vi "getTagfromId.vi"(10 "ID":dbl, 11 "PipelineResult":T7={"TargetCount"=0, "Latency_MilliSec"=0.0, "Targets"=[], "TimeStampSec"=0.0, "PhotonMultiTargetPNPResult"={"PhotonPNPResult"={"IsPresent"=FALSE, "bestReprojErr"=0.0, "altReprojErr"=0.0, "ambiguity"=0.0, "Best"={"TRANSLATION3D"={"X"=0.0, "Y"=0.0, "Z"=0.0}, "ROTATION3D"={"Q_quaternion"={"R"=1.0, "V"=[0.0, 0.0, 0.0]}}, "XF"=FALSE}, "Alt"={"TRANSLATION3D"={"X"=0.0, "Y"=0.0, "Z"=0.0}, "ROTATION3D"={"Q_quaternion"={"R"=1.0, "V"=[0.0, 0.0, 0.0]}}, "XF"=FALSE}}, "FiducialIDsUsed"=[]}} {"PhotonMultiTargetPNPResult"."PhotonPNPResult"."Alt"."TRANSLATION3D"."Z" format="%14.3f"; "PhotonMultiTargetPNPResult"."PhotonPNPResult"."Alt"."TRANSLATION3D"."Y" format="%14.3f"; "PhotonMultiTargetPNPResult"."PhotonPNPResult"."Alt"."TRANSLATION3D"."X" format="%14.3f"; "PhotonMultiTargetPNPResult"."PhotonPNPResult"."Best"."TRANSLATION3D"."Z" format="%14.3f"; "PhotonMultiTargetPNPResult"."PhotonPNPResult"."Best"."TRANSLATION3D"."Y" format="%14.3f"; "PhotonMultiTargetPNPResult"."PhotonPNPResult"."Best"."TRANSLATION3D"."X" format="%14.3f"; "Targets"."AltCameraToTarget"."TRANSLATION3D"."Z" format="%14.3f"; "Targets"."AltCameraToTarget"."TRANSLATION3D"."Y" format="%14.3f"; "Targets"."AltCameraToTarget"."TRANSLATION3D"."X" format="%14.3f"; "Targets"."BestCameraToTarget"."TRANSLATION3D"."Z" format="%14.3f"; "Targets"."BestCameraToTarget"."TRANSLATION3D"."Y" format="%14.3f"; "Targets"."BestCameraToTarget"."TRANSLATION3D"."X" format="%14.3f"}) -> (3 "PhotonTrackedTarget":T1={"Yaw"=0.0, "Pitch"=0.0, "Area"=0.0, "Skew"=0.0, "MinAreaRectCorners"=[], "BestCameraToTarget"={"TRANSLATION3D"={"X"=0.0, "Y"=0.0, "Z"=0.0}, "ROTATION3D"={"Q_quaternion"={"R"=1.0, "V"=[0.0, 0.0, 0.0]}}, "XF"=FALSE}, "FiiducialId"=0, "AltCameraToTarget"={"TRANSLATION3D"={"X"=0.0, "Y"=0.0, "Z"=0.0}, "ROTATION3D"={"Q_quaternion"={"R"=1.0, "V"=[0.0, 0.0, 0.0]}}, "XF"=FALSE}, "PoseAmbiguity"=0.0, "DetectedCorners"=[]} {"AltCameraToTarget"."TRANSLATION3D"."Z" format="%14.3f"; "AltCameraToTarget"."TRANSLATION3D"."Y" format="%14.3f"; "AltCameraToTarget"."TRANSLATION3D"."X" format="%14.3f"; "BestCameraToTarget"."TRANSLATION3D"."Z" format="%14.3f"; "BestCameraToTarget"."TRANSLATION3D"."Y" format="%14.3f"; "BestCameraToTarget"."TRANSLATION3D"."X" format="%14.3f"})   [LabVIEW 2023]
uses:
  <vilib>/Rock Robotics/WPI/ThirdParty/PhotonVisionLib/TypeDef/PhotonPipelineResultType.ctl
  <vilib>/Rock Robotics/WPI/ThirdParty/PhotonVisionLib/TypeDef/PhotonTrackedTargetType.ctl
  <vilib>/Rock Robotics/WPI/ThirdParty/PhotonVisionLib/TypeDef/TargetCornerType.ctl
  <vilib>/Rock Robotics/WPI/ThirdParty/JAS_Junk/TrajLib/TypeDef/TRANSFORM3D.ctl
  <vilib>/Rock Robotics/WPI/ThirdParty/JAS_Junk/TrajLib/TypeDef/TRANSLATION3D.ctl
  <vilib>/Rock Robotics/WPI/ThirdParty/JAS_Junk/TrajLib/TypeDef/ROTATION3D.ctl
  <vilib>/Rock Robotics/WPI/ThirdParty/JAS_Junk/TrajLib/TypeDef/QUATERNION.ctl
  <vilib>/Rock Robotics/WPI/ThirdParty/PhotonVisionLib/TypeDef/PhotonMultiTargetPNPResultType.ctl
  <vilib>/Rock Robotics/WPI/ThirdParty/PhotonVisionLib/TypeDef/PhotonPNPResultType.ctl
  <vilib>/Rock Robotics/WPI/ThirdParty/PhotonVisionLib/PhotonVisionLib.lvlib
  <vilib>/Rock Robotics/WPI/ThirdParty/JAS_Junk/TrajLib/Trajectory_Library.lvlib
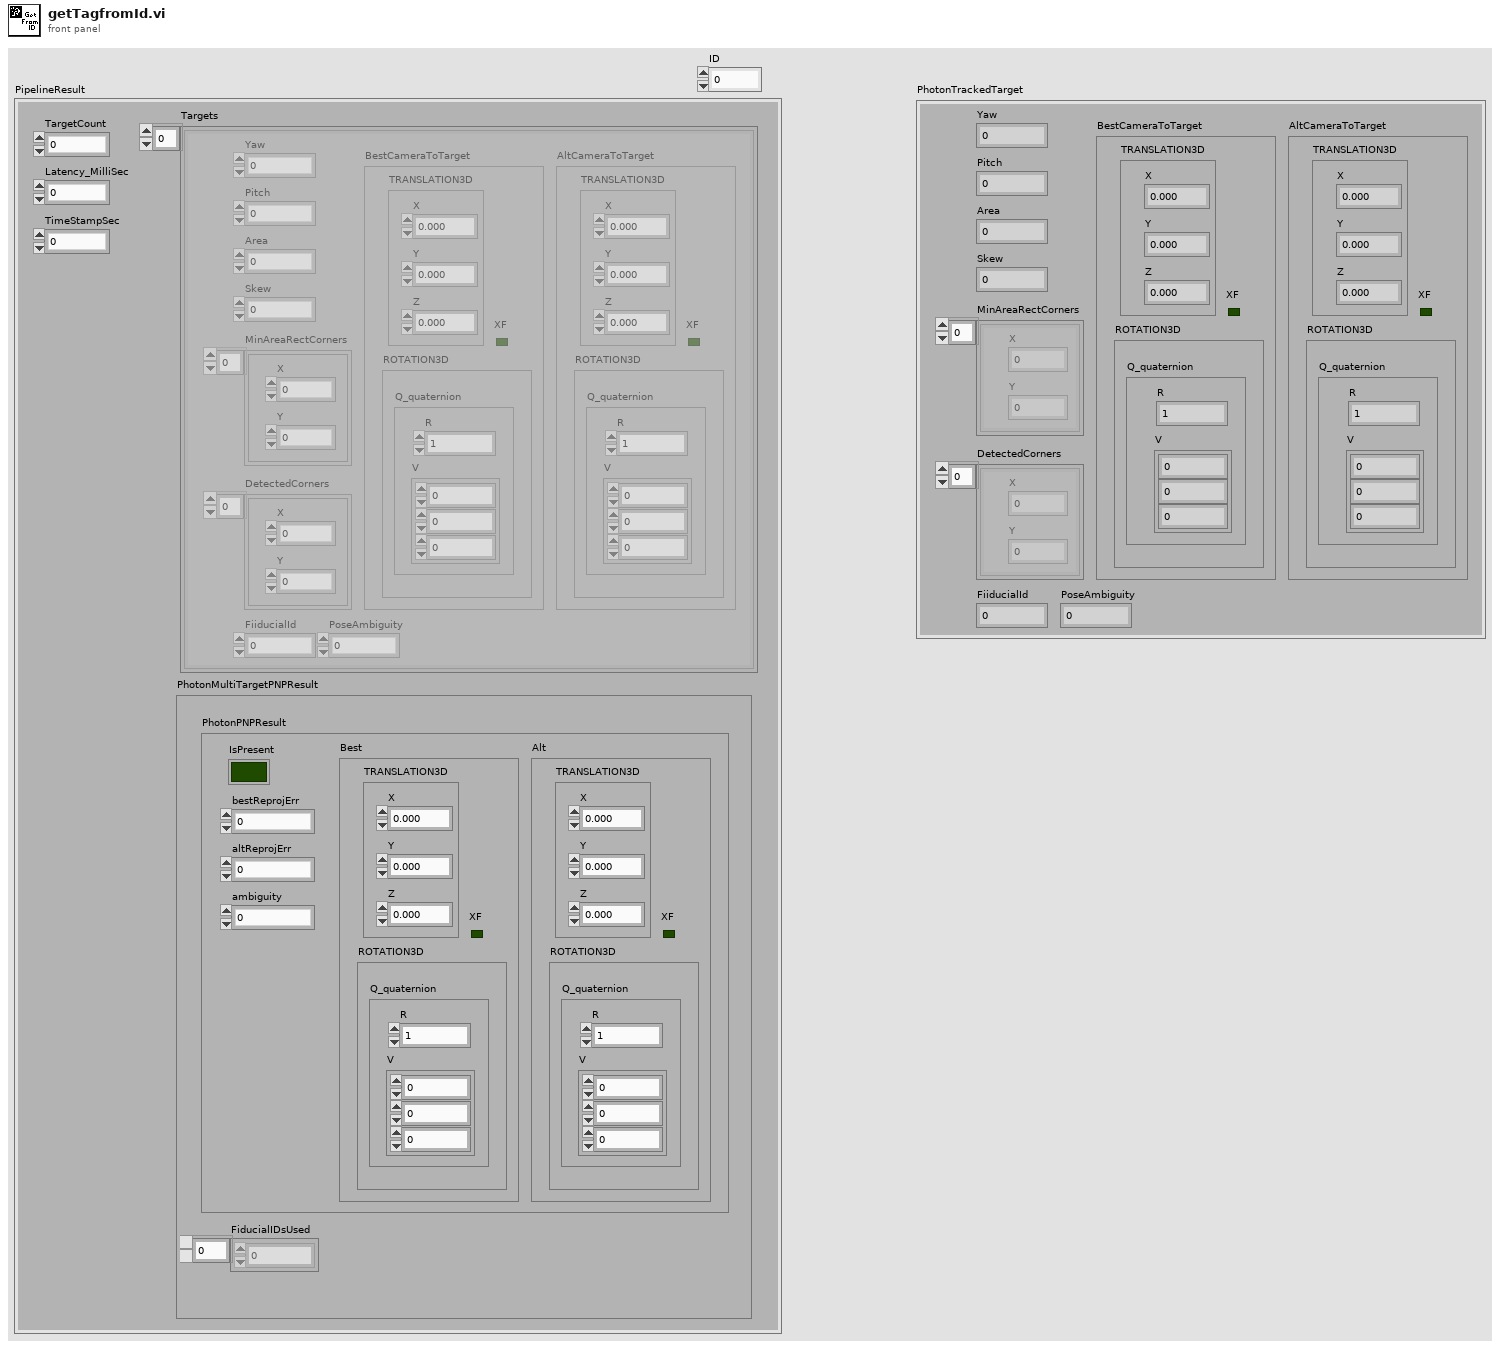
[diagram p1: front panel]
types:
  T1 = typedef "PhotonVisionLib.lvlib/PhotonTrackedTargetType.ctl" = cluster{"Yaw":dbl, "Pitch":dbl, "Area":dbl, "Skew":dbl, "MinAreaRectCorners":T2[], "BestCameraToTarget":T3, "FiiducialId":i32, "AltCameraToTarget":T3, "PoseAmbiguity":dbl, "DetectedCorners":T2[]}
  T2 = typedef "PhotonVisionLib.lvlib/TargetCornerType.ctl" = cluster{"X":dbl, "Y":dbl}
  T3 = typedef "Trajectory_Library.lvlib/TRANSFORM3D.ctl" = cluster{"TRANSLATION3D":T4, "ROTATION3D":T5, "XF":bool}
  T4 = typedef "Trajectory_Library.lvlib/TRANSLATION3D.ctl" = cluster{"X":dbl, "Y":dbl, "Z":dbl}
  T5 = typedef "Trajectory_Library.lvlib/ROTATION3D.ctl" = cluster{"Q_quaternion":T6}
  T6 = typedef "Trajectory_Library.lvlib/QUATERNION.ctl" = cluster{"R":dbl, "V":dbl[]}
  T7 = typedef "PhotonVisionLib.lvlib/PhotonPipelineResultType.ctl" = cluster{"TargetCount":i32, "Latency_MilliSec":dbl, "Targets":T1[], "TimeStampSec":dbl, "PhotonMultiTargetPNPResult":T8}
  T8 = typedef "PhotonVisionLib.lvlib/PhotonMultiTargetPNPResultType.ctl" = cluster{"PhotonPNPResult":T9, "FiducialIDsUsed":i16[]}
  T9 = typedef "PhotonVisionLib.lvlib/PhotonPNPResultType.ctl" = cluster{"IsPresent":bool, "bestReprojErr":dbl, "altReprojErr":dbl, "ambiguity":dbl, "Best":T3, "Alt":T3}
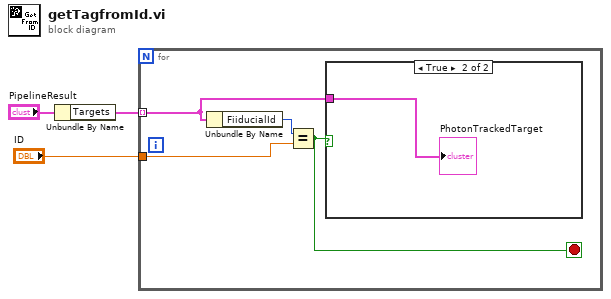
[diagram p0: block diagram]
diagram:
  n1 = Unbundle By Name("PipelineResult") -> ("Targets"=w2:T1[])
  n2 = for {
    tunnel: w2 -> [w5] mode=indexing
    tunnel: "ID" -> [w6]
    stop <- w4 stop-if-true
    n3 = Unbundle By Name(w5) -> ("FiiducialId"=w7:i32)
    n4 = Equal?(x=w7, y=w6) -> (x = y?=w4:bool)
    n5 = case shown="True" w4 {
      tunnel: w5 -> [_ w8]
      frame False {
      }
      frame True {
        "PhotonTrackedTarget" <- w8
      }
    }
  }
